vi "OpenCV UnsharpMask.vi"(6 "Threshold":sgl, 7 "Amount":sgl, 8 "error in (no error)":errorcluster, 9 "Radius":sgl, 10 "Image Dst":T1, 11 "Image Src":T1) -> (0 "error out":errorcluster, 3 "Image Dst Out":T1)   [LabVIEW 2023]
uses:
  <vilib>/vision/Image Controls.llb/IMAQ Image.ctl
  build/OpenCVWrapper.dll
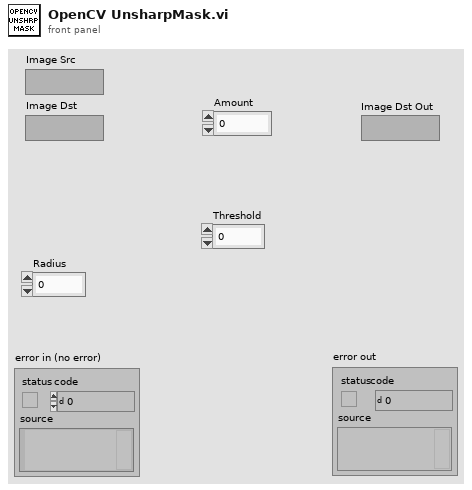
[diagram p1: front panel]
types:
  T1 = typedef "IMAQ Image.ctl" = refnum<image>
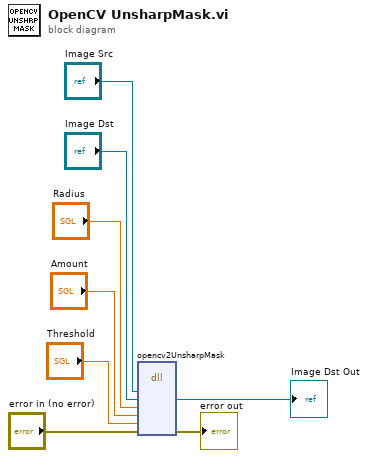
[diagram p0: block diagram]
diagram:
  n1 = dll-call lib="D:/XRay Experiments/OpenCVWrapper/build/OpenCVWrapper.dll" fn="opencv2UnsharpMask"("src"="Image Src", "dst"="Image Dst", "Radius"="Radius", "Amount"="Amount", "Threshold"="Threshold", "error"="error in (no error)") -> ("dst"=→"Image Dst Out":T1, "error"=→"error out":errorcluster)  [unwired: 8 in, 2 out]
